vi "Proton's momentum.vi"(10 "Starting Velocity":dbl) -> (2 "Momentum":dbl)   [LabVIEW 2020]
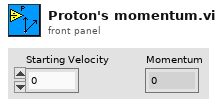
[diagram p1: front panel]
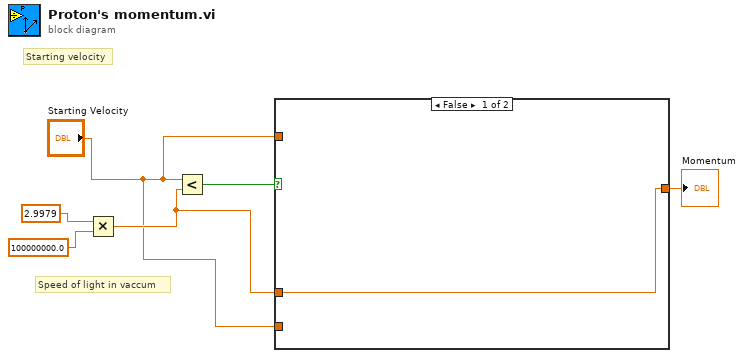
[diagram p0: block diagram]
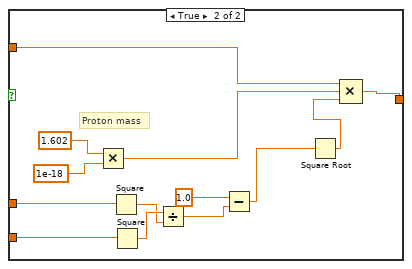
[diagram p2: hidden frame]
diagram:
  # "Speed of light in vaccum"
  # "Starting velocity"
  n1 = Multiply(x=2.9979, y=100000000.0) -> (x*y=w3:dbl)
  n2 = Less?(x="Starting Velocity", y=w3) -> (x < y?=w4:bool)
  n3 = case shown="False" w4 {
    tunnel: "Starting Velocity" -> [_ w17]
    tunnel: w3 -> [w7 w15]
    tunnel: "Starting Velocity" -> [_ w14]
    tunnel: [w7 w8] -> w1
    frame False {
    }
    frame True {
      # "Proton mass"
      n4 = Multiply(x=1.602, y=1e-18) -> (x*y=w18:dbl)
      n5 = Square(x=w15) -> (x^2=w12:dbl)
      n6 = Square(x=w14) -> (x^2=w13:dbl)
      n7 = Divide(x=w13, y=w12) -> (x/y=w11:dbl)
      n8 = Subtract(x=1.0, y=w11) -> (x-y=w10:dbl)
      n9 = Square Root(x=w10) -> (sqrt(x)=w9:dbl)
      n10 = Compound Arithmetic op=MULTIPLY(w17, w18, w9) -> (w8:dbl)
    }
  }
  "Momentum" <- w1
